vi "GetExternalInterfaces.vi"(8 "ErrorIn":errorcluster, 11 "ReferenceIn":refnum<class "UserManager.lvclass">) -> (0 "ErrorOut":errorcluster, 2 "ExternalInterfaces":T1[](array[typedef]), 3 "ReferenceOut":refnum<class "UserManager.lvclass">)   [LabVIEW 2021, in "UserMananger.lvlib" / "UserManager.lvclass"]
uses:
  UserManager.lvclass
  Library_TAF_Support/ClusterArrayConversion/BundledArray.ctl
  c918bead-a22c-460a-a6f4-f95520c4e6a6.vi
  c918bead-a22c-460a-a6f4-f95520c4e6a6.vi/e733eca7-9823-4359-8665-3b184f9a7377.vi
  <vilib>/Utility/Data Type/Get Cluster Information.vi
  <vilib>/Utility/Data Type/Get Type Information.vi
  UserManager.lvclass/UserManager.ctl
  Library_TAF_Support/ClusterArrayConversion/ClusterArrayConversion.lvlib
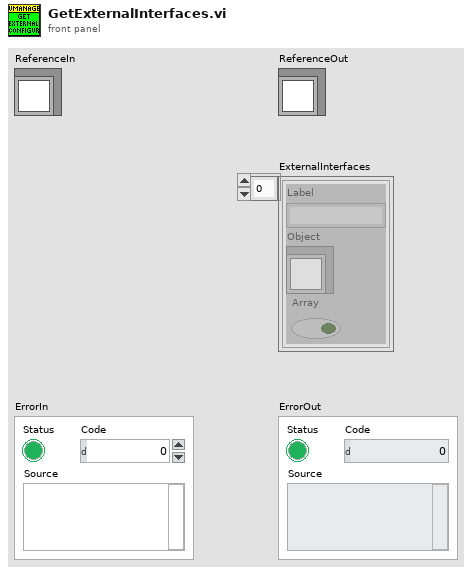
[diagram p1: front panel]
types:
  T1 = typedef "ClusterArrayConversion.lvlib/BundledArray.ctl" = cluster{"Label":string, "Object":refnum<class>, "Array":bool}
  T2 = typedef "UserMananger.lvlib/UserManager.lvclass/ObjectAttributes.ctl" = cluster{"Interfaces":cluster{"ActivationUpdated":refnum<class "IAuthorizationUpdated.lvclass">}, "Locals":cluster{"MainGUIActive":refnum<queue>, "Evaluations":cluster{"Label":string, "Value":string}[]}, "Persistent":cluster{"Dummy":bool}}
  T3 = cluster{"ActivationUpdated":refnum<class "IAuthorizationUpdated.lvclass">}
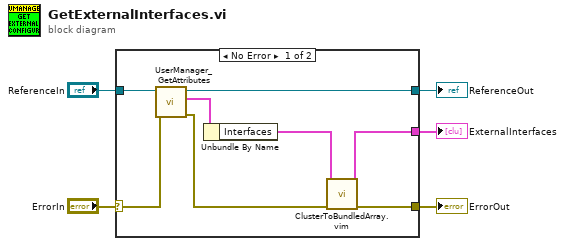
[diagram p0: block diagram]
diagram:
  n1 = case shown="No Error" "ErrorIn" {
    selector: "ErrorIn" -> [w13 w15]
    tunnel: [w11 w15] -> w4
    tunnel: [w8 w14] -> w2
    tunnel: "ReferenceIn" -> [w9 w14]
    tunnel: [w6 _] -> w1
    frame No Error {
      n2 = call "UserManager_GetAttributes.vi"("ErrorIn"=w13, "ReferenceIn"=w9) -> ("ErrorOut"=w12:errorcluster, "Data"=w10:T2, "ReferenceOut"=w8:refnum<class "UserManager.lvclass">)  [unwired: 6 in, 1 out]
      n3 = Unbundle By Name(w10) -> ("Interfaces"=w7:T3)
      n4 = call "ClusterToBundledArray.vim"("ErrorIn"=w12, "Interfaces"=w7) -> ("ErrorOut"=w11:errorcluster, "BundeledLabels"=w6:T1[])  [unwired: 8 in]
    }
    frame Error {
    }
  }
  "ErrorOut" <- w4
  "ReferenceOut" <- w2
  "ExternalInterfaces" <- w1
